vi "generate default line.vi"(8 "error in":errorcluster, 10 "last line item":T1, 11 "operations table":refnum<vi>) -> (0 "error out":errorcluster, 2 "line item in":T1)   [LabVIEW 2013, in "Scan Engine editor node.lvclass"]
uses:
  Scan Engine editor node.lvclass
  table line.ctl
  <vilib>/NI/Tag Bus Module Framework/channel/TBM channel.lvclass
  <vilib>/NI/Tag Bus/tag/tag descriptor.lvclass/tag descriptor.ctl
  <vilib>/NI/Tag Bus Module Framework/channel/TBM channel.lvclass/TBM channel.ctl
  <vilib>/NI/Tag Bus/tag/Data Type.ctl
  permissions.ctl
  <vilib>/NI/Tag Bus/tag/read data type.vi
  <vilib>/NI/Tag Bus Module Framework/channel/Read channel classification.vi
  <vilib>/NI/Tag Bus/tag/tag descriptor.lvclass
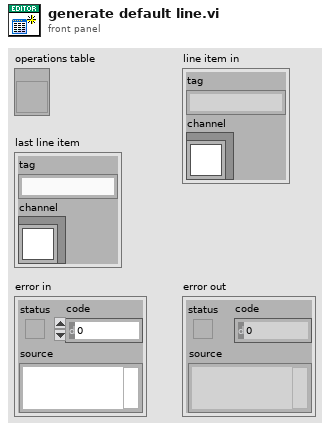
[diagram p1: front panel]
types:
  T1 = typedef "Scan Engine editor node.lvclass/table line.ctl" = cluster{"tag":string, "channel":refnum<class "TBM channel.lvclass">}
  T2 = typedef "tag bus.lvlib/tag descriptor.lvclass/Data Type.ctl" = enum16{"Double", "Single", "I64", "I32", "I16", "I8", "U64", "U32", "U16", "U8", "Boolean", "String", "Array of Double", "Array of Single", "Array of I64", "Array of I32", "Array of I16", "Array of I8", "Array of U64", "Array of U32", "Array of U16", "Array of U8", "Array of Boolean", "Array of String"}
  T3 = typedef "TBM channel.lvclass/channel classification.ctl" = enum16{"input data", "output data", "processing parameter", "processing result"}
  T4 = typedef "Scan Engine editor node.lvclass/permissions.ctl" = enum32{"Read from HW", "Write to HW"}
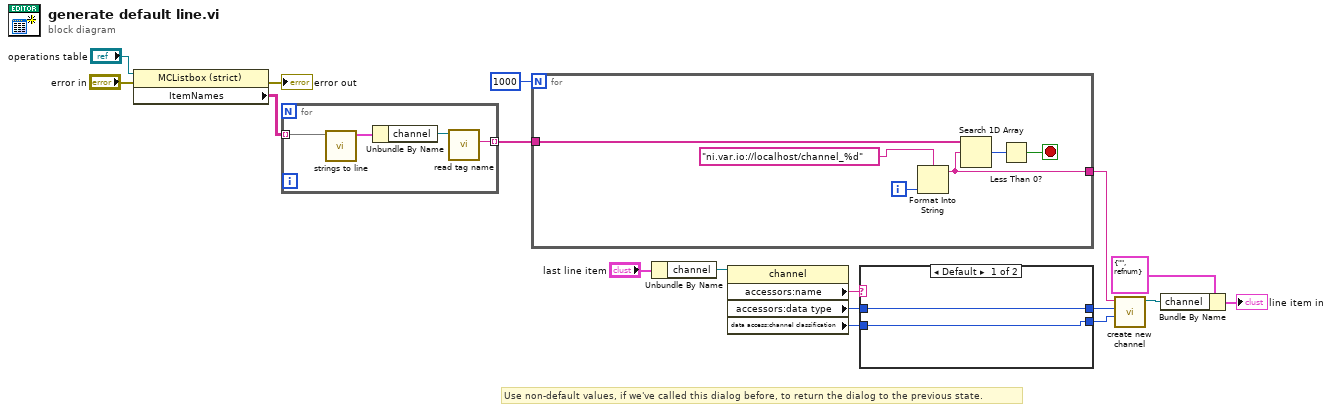
[diagram p0: block diagram]
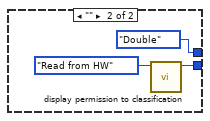
[diagram p2: hidden frame]
diagram:
  # "Use non-default values, if we've called this dialog before, to return the dialog to the previous state."
  n1 = property class="MCListbox (strict)"(reference="operations table", error in="error in") -> (error out=→"error out":errorcluster, "ItemNames"=w14:string[][])  [unwired: 1 out]
  n2 = for {
    tunnel: w14 -> [w21] mode=indexing
    tunnel: [w18] -> w12 mode=indexing
    n3 = call "strings to line.vi"("strings"=w21) -> ("line"=w20:T1)  [unwired: 10 in]
    n4 = Unbundle By Name(w20) -> ("channel"=w19:refnum<class "TBM channel.lvclass">)
    n5 = call <vilib>:"read tag name.vi"("system tag in"=w19) -> ("name"=w18:string)  [unwired: 8 in, 2 out]
  }
  n6 = for {
    N: 1000 -> [_]
    tunnel: w12 -> [w25]
    tunnel: [w22] -> w11
    i -> [w27]
    stop <- w23 stop-if-true
    n7 = Format Into String(format string="ni.var.io://localhost/channel_%d", w27) -> (resulting string=w22:string)  [unwired: 2 in, 1 out]
    n8 = Search 1D Array(1D array=w25, element=w22) -> (index of element=w24:i32)  [unwired: 1 in]
    n9 = Less Than 0?(x=w24) -> (x < 0?=w23:bool)
  }
  n10 = Unbundle By Name("last line item") -> ("channel"=w4:refnum<class "TBM channel.lvclass">)
  n11 = property class="channel"(reference=w4) -> ("accessors:name"=w3:string, "accessors:data type"=w2:T2, "data access:channel classification"=w1:T3)  [unwired: 1 in, 2 out]
  n12 = case shown="Default" w3 {
    tunnel: [w29 Data_Type."Double" ("data type")] -> w10
    tunnel: [w28 w30] -> w9
    tunnel: w2 -> [w29 _]
    tunnel: w1 -> [w28 _]
    frame Default {
    }
    frame "" {
      n13 = call "display permission to classification.vi"("display permissions"=permissions."Read from HW") -> ("channel classification"=w30:T3)  [unwired: 10 in]
    }
  }
  n14 = call <vilib>:"create new channel.vi"("channel classification"=w9, "data type"=w10, "channel name"=w11) -> ("channel"=w6:refnum<class "TBM channel.lvclass">)  [unwired: 8 in]
  n15 = Bundle By Name(cluster=T1 {"tag"="", "channel"=refnum} ("line item in 2"), "channel"=w6) -> (→"line item in":T1)
